vi "FILE PATH.vi"() -> ()   [LabVIEW 2015]
uses:
  <vilib>/Utility/config.llb/Write Key (String).vi
  <vilib>/Utility/config.llb/NI_LVConfig.lvlib
panel:
  in  "Enter the path and the name of the ini file":path
  out "The directory":string
  out "The folder of the VI":string
  out "The VI":string
  in  "Choose the path of the VI":path
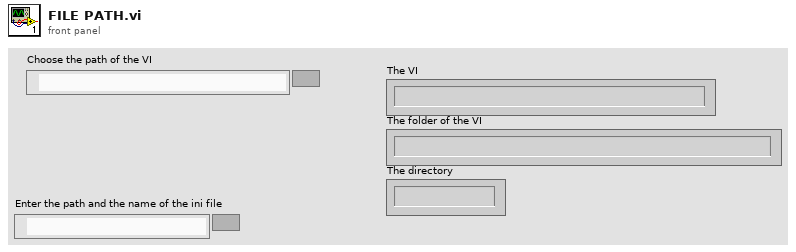
[diagram p1: front panel]
types:
  T1 = typedef "NI_LVConfig.lvlib/Config Data RefNum.ctl" = refnum<k1>
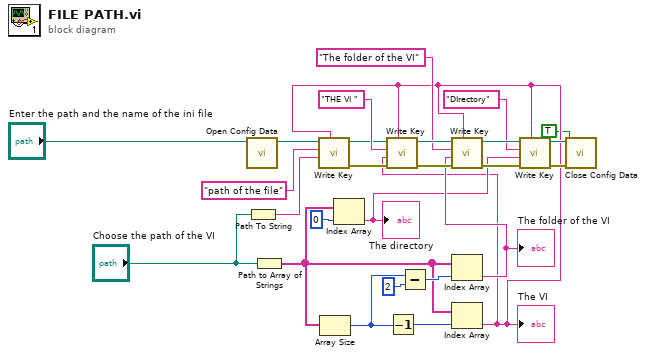
[diagram p0: block diagram]
diagram:
  n1 = call <vilib>:"Open Config Data.vi"("configuration file path"="Enter the path and the name of the ini file") -> ("refnum"=w7:T1)  [unwired: 8 in, 2 out]
  n2 = Path To String(path="Choose the path of the VI") -> (string=w6:string)
  n3 = Path to Array of Strings(0:"Choose the path of the VI") -> (2:w9:string[])  [unwired: 1 out]
  n4 = Array Size(array=w9) -> (size(s)=w23:i32)
  n5 = Index Array(array=w9, index=0) -> (element=w4:string)
  "The directory" <- w4
  n6 = Decrement(x=w23) -> (x-1=w24:i32)
  n7 = Subtract(x=w23, y=2) -> (x-y=w21:i32)
  n8 = Index Array(array=w9, index=w21) -> (element=w5:string)
  "The folder of the VI" <- w5
  n9 = Index Array(array=w9, index=w24) -> (element=w2:string)
  "The VI" <- w2
  n10 = call-poly <vilib>:"Write Key.vi"("section"=w2, "value"=w6, "key"="path of the file", "refnum"=w7) -> ("error out"=w8:errorcluster, "refnum out"=w13:T1)  [unwired: 5 in, 1 out]
  n11 = call-poly <vilib>:"Write Key.vi"("section"=w2, "error in (no error)"=w8, "value"=w2, "key"="THE VI ", "refnum"=w13) -> ("error out"=w17:errorcluster, "refnum out"=w20:T1)  [unwired: 4 in, 1 out]
  n12 = call-poly <vilib>:"Write Key.vi"("section"=w2, "error in (no error)"=w17, "value"=w5, "key"="The folder of the VI", "refnum"=w20) -> ("error out"=w16:errorcluster, "refnum out"=w19:T1)  [unwired: 4 in, 1 out]
  n13 = call-poly <vilib>:"Write Key.vi"("section"=w2, "error in (no error)"=w16, "value"=w4, "key"="DIrectory", "refnum"=w19) -> ("error out"=w15:errorcluster, "refnum out"=w18:T1)  [unwired: 4 in, 1 out]
  n14 = call <vilib>:"Close Config Data.vi"("error in (no error)"=w15, "write file if changed (T)"=TRUE, "refnum"=w18) -> ()  [unwired: 7 in, 2 out]
